vi "load.vi"(8 "error in (no error)":errorcluster, 9 "page":i32, 10 "Path":path, 11 "Image in":refnum<class "Image.lvclass">) -> (0 "error out":errorcluster, 1 "Path out":path, 2 "cancelled?":bool, 3 "Image out":refnum<class "Image.lvclass">)   [LabVIEW 2010, in "Image.lvclass"]
uses:
  Image.lvclass
  storage_mode.ctl
  <vilib>/regexp/Match Regular Expression.xnode
  XMLElement/XMLElement/XMLElement.lvclass
  enumerations/unit.ctl
  ErrorController/ErrorController/class_data.vi
  libraries/TIFFManagement/TIFFManagement.lvlib
  ErrorController/ErrorController/ErrorController.lvclass
panel:
  out "Intensity Graph":u32[][](graph)
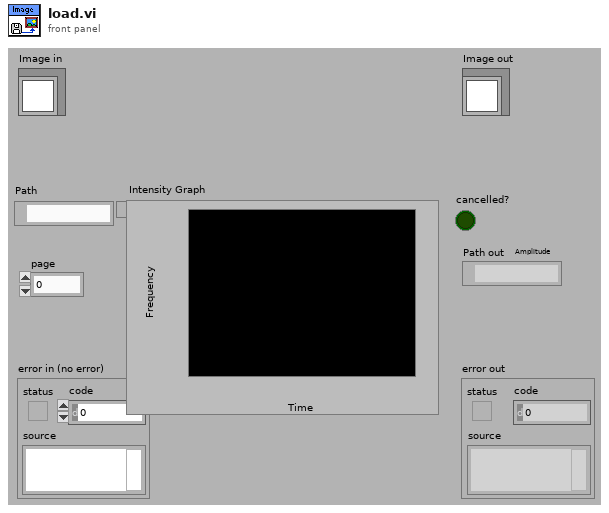
[diagram p1: front panel]
types:
  T1 = typedef "Image.lvclass/storage_mode.ctl" = enum16{"RAM", "disk"}
  T2 = typedef "Image Type" = u32
  T3 = typedef "IMAQ Image.ctl" = refnum<image>
  T4 = typedef "Image.lvclass/unit.ctl" = enum16{"um", "s"}
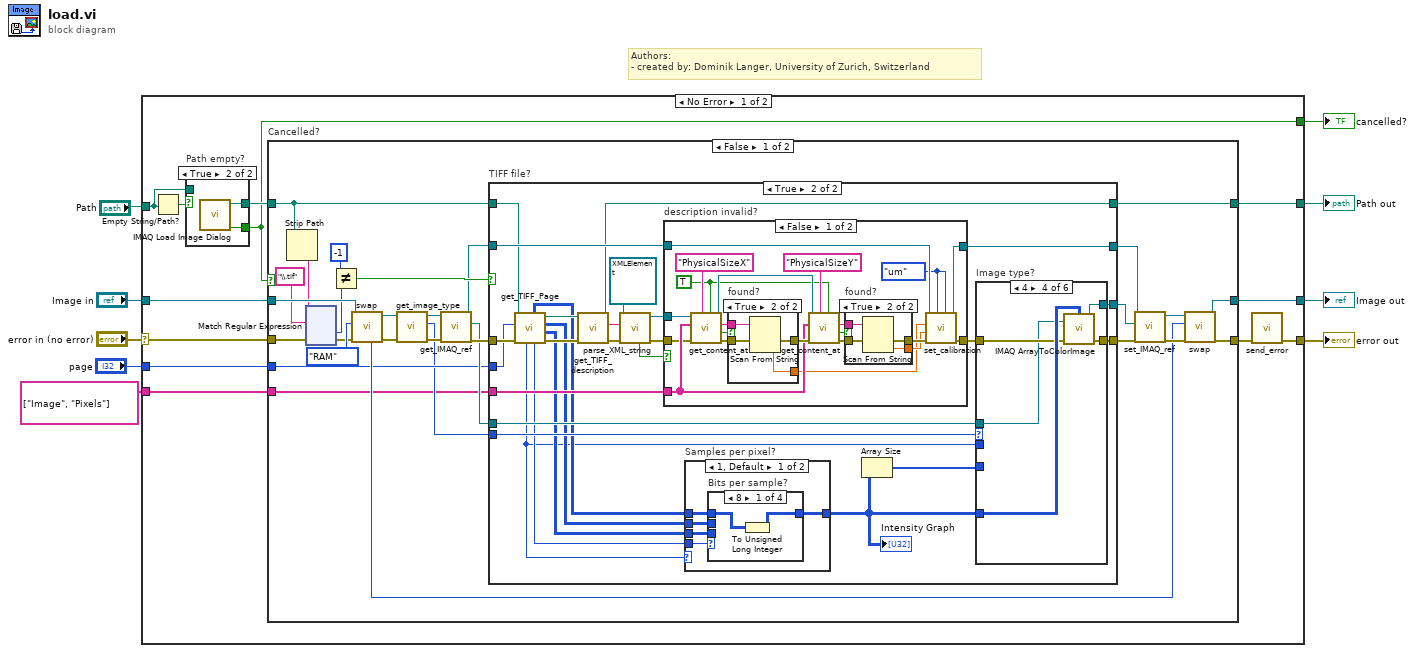
[diagram p0: block diagram]
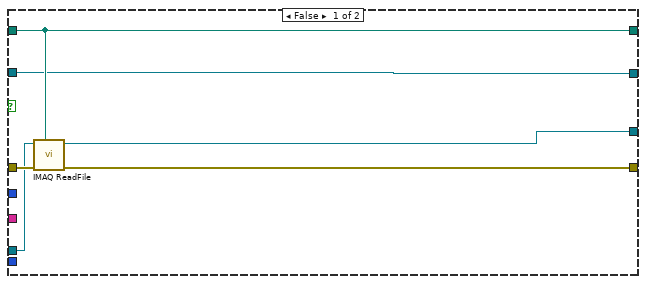
[diagram p2: hidden frame]
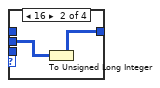
[diagram p3: hidden frame]
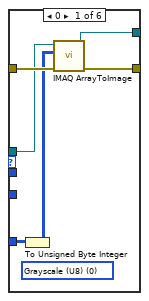
[diagram p10: hidden frame]
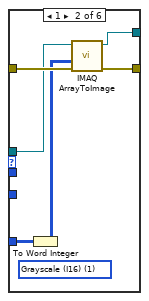
[diagram p11: hidden frame]
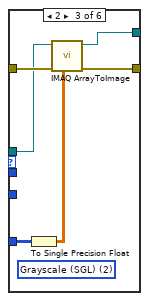
[diagram p12: hidden frame]
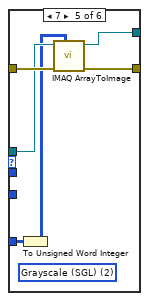
[diagram p13: hidden frame]
diagram:
  # "Authors: \n- created by: Dominik Langer, University of Zurich, Switzerland"
  n1 = case shown="No Error" "error in (no error)" {
    selector: "error in (no error)" -> [w18 w276]
    tunnel: [w11 w276] -> w8
    tunnel: [w20 w275] -> w6
    tunnel: "Image in" -> [w19 w275]
    tunnel: "Path" -> [w17 _]
    tunnel: [w15 _] -> w5
    tunnel: [w14 _] -> w4
    tunnel: "page" -> [w13 _]
    tunnel: string[] ["Image", "Pixels"] ("key chain") -> [w12 _]
    frame No Error {
      n2 = Empty String/Path?(string/path=w17) -> (empty?=w16:bool)
      n3 = case "Path empty?" shown="True" w16 {
        tunnel: [w272 w274] -> w21
        tunnel: w17 -> [w272 _]
        tunnel: [_ w273] -> w15
        frame False {
        }
        frame True {
          n4 = call "IMAQ Load Image Dialog"() -> ("Cancelled?"=w273:bool, "Path"=w274:path)  [unwired: 7 in, 3 out]
        }
      }
      n5 = case "Cancelled?" shown="False" w15 {
        tunnel: w21 -> [w47 _]
        tunnel: [w50 w271] -> w10
        tunnel: [w49 w270] -> w20
        tunnel: w19 -> [w48 w270]
        tunnel: w18 -> [w27 w271]
        tunnel: [w36 _] -> w14
        tunnel: w13 -> [w35 _]
        tunnel: w12 -> [w22 _]
        frame False {
          n6 = Strip Path(path=w47) -> (name=w25:string)  [unwired: 1 out]
          n7 = xnode "Match Regular Expression"("input string"=w25, "regular expression"="\\.tif", "error in"=w27) -> ("offset past match"=w23:i32, "error out"=w26:errorcluster)  [unwired: 3 in, 3 out]
          n8 = Not Equal?(x=-1, y=w23) -> (x != y?=w37:bool)
          n9 = call-dynamic "swap.vi"("error in (no error)"=w26, "storage type target"=storage_mode."RAM", "Image in"=w48) -> ("error out"=w34:errorcluster, "Image out"=w33:refnum<class "Image.lvclass">, "previous storage mode"=w39:T1)  [unwired: 6 out]
          n10 = call-dynamic "get_image_type.vi"("error in (no error)"=w34, "Image.lvclass in"=w33) -> ("error out"=w32:errorcluster, "Image Type"=w30:T2, "Image.lvclass out"=w31:refnum<class "Image.lvclass">)  [unwired: 6 in, 1 out]
          n11 = call-dynamic "get_IMAQ_ref.vi"("error in (no error)"=w32, "Image.lvclass in"=w31) -> ("error out"=w43:errorcluster, "Image"=w42:T3, "Image.lvclass out"=w29:refnum<class "Image.lvclass">)  [unwired: 7 out]
          n12 = case "TIFF file?" shown="True" w37 {
            tunnel: w47 -> [w163 w186]
            tunnel: [w167 w189] -> w45
            tunnel: [w166 w194] -> w44
            tunnel: w43 -> [w165 w187]
            tunnel: w42 -> [w164 w193]
            tunnel: [w163 w182] -> w36
            tunnel: w35 -> [_ w185]
            tunnel: w30 -> [_ w192]
            tunnel: w29 -> [w162 w191]
            tunnel: [w162 w190] -> w28
            tunnel: w22 -> [_ w181]
            frame False {
              n13 = call "IMAQ ReadFile"("File Path"=w163, "error in (no error)"=w165, "Image"=w164) -> ("error out"=w167:errorcluster, "Image Out"=w166:T3)  [unwired: 2 in, 5 out]
            }
            frame True {
              n14 = call "get_TIFF_Page.vi"("error in (no error)"=w187, "page"=w185, "path in"=w186) -> ("error out"=w184:errorcluster, "data 32bit"=w178:u32[][], "data 16bit"=w180:u16[][], "path out"=w183:path, "bits per sample"=w177:u16, "data 8bit"=w179:u8[][], "samples per pixel"=w176:i32)  [unwired: 2 in]
              n15 = call "get_TIFF_description.vi"("error in (no error)"=w184, "path in"=w183) -> ("error out"=w172:errorcluster, "description"=w173:string, "path out"=w182:path)  [unwired: 6 in, 1 out]
              n16 = call "parse_XML_string.vi"("error in (no error)"=w172, "XML string"=w173, "Element in"=refnum<class "XMLElement.lvclass"> refnum ("XMLElement.lvclass")) -> ("error out"=w171:errorcluster, "Element out"=w168:refnum<class "XMLElement.lvclass">, "header empty or invalid XML?"=w169:bool)  [unwired: 6 in]
              n17 = case "description invalid?" shown="False" w169 {
                tunnel: w191 -> [w226 w238]
                tunnel: [w225 w238] -> w190
                tunnel: [w223 w237] -> w188
                tunnel: w171 -> [w207 w237]
                tunnel: w181 -> [w214 _]
                tunnel: w168 -> [w206 _]
                frame False {
                  w211 = TRUE
                  w224 = unit."um" ("x unit")
                  n18 = call "get_content_at.vi"("ignore IDs"=w211, "attribute name"="PhysicalSizeX", "error in (no error)"=w207, "key chain"=w214, "Element in"=w206) -> ("error out"=w221:errorcluster, "found?"=w210:bool, "string"=w219:string, "Element out"=w222:refnum<class "XMLElement.lvclass">)  [unwired: 3 in]
                  n19 = case "found?" shown="True" w210 {
                    tunnel: w221 -> [w232 w236]
                    tunnel: [w232 w235] -> w220
                    tunnel: [_ w234] -> w209
                    tunnel: w219 -> [_ w233]
                    frame False {
                    }
                    frame True {
                      n20 = Scan From String(input string=w233, error in=w236) -> (error out=w235:errorcluster, output 1=w234:dbl)  [unwired: 3 in, 2 out]
                    }
                  }
                  n21 = call "get_content_at.vi"("ignore IDs"=w211, "attribute name"="PhysicalSizeY", "error in (no error)"=w220, "key chain"=w214, "Element in"=w222) -> ("error out"=w218:errorcluster, "found?"=w208:bool, "string"=w216:string)  [unwired: 3 in, 1 out]
                  n22 = case "found?" shown="True" w208 {
                    tunnel: w218 -> [w227 w231]
                    tunnel: [w227 w230] -> w217
                    tunnel: w216 -> [_ w229]
                    tunnel: [_ w228] -> w215
                    frame False {
                    }
                    frame True {
                      n23 = Scan From String(input string=w229, error in=w231) -> (error out=w230:errorcluster, output 1=w228:dbl)  [unwired: 3 in, 2 out]
                    }
                  }
                  n24 = call "set_calibration.vi"("y unit"=w224, "x unit"=w224, "error in (no error)"=w217, "y"=w215, "x"=w209, "Image in"=w226) -> ("error out"=w223:errorcluster, "Image out"=w225:refnum<class "Image.lvclass">)  [unwired: 4 in]
                }
                frame True {
                }
              }
              n25 = case "Samples per pixel?" shown="1, Default" w176 {
                tunnel: w180 -> [w195 _]
                tunnel: w179 -> [w198 _]
                tunnel: w178 -> [w196 w205]
                tunnel: [w197 w205] -> w175
                tunnel: w177 -> [w199 _]
                frame 1, Default {
                  n26 = case "Bits per sample?" shown="8" w199 {
                    tunnel: w198 -> [w201 _ _ _]
                    tunnel: [w200 w203 w204 _] -> w197
                    tunnel: w196 -> [_ _ w204 _]
                    tunnel: w195 -> [_ w202 _ _]
                    frame 8 {
                      n27 = To Unsigned Long Integer(number=w201) -> (unsigned 32bit integer=w200:u32[][])
                    }
                    frame 16 {
                      n28 = To Unsigned Long Integer(number=w202) -> (unsigned 32bit integer=w203:u32[][])
                    }
                    frame 32 {
                    }
                    frame Default {
                    }
                  }
                }
                frame 3 {
                }
              }
              "Intensity Graph" <- w175
              n29 = Array Size(array=w175) -> (size(s)=w174:i32[])
              n30 = case "Image type?" shown="4" w192 {
                tunnel: w188 -> [w243 w250 w255 w260 w267 w268]
                tunnel: [w241 w249 w252 w258 w266 w268] -> w189
                tunnel: w175 -> [w244 w246 w256 w261 w263 _]
                tunnel: [w240 w248 w251 w257 w265 w269] -> w194
                tunnel: w193 -> [w242 w247 w254 w259 w264 w269]
                tunnel: w176 -> [_ _ _ _ _ _]
                tunnel: w174 -> [_ _ _ _ _ _]
                frame 0 {
                  (unwired) T2 0 items=["Grayscale (U8)", "Grayscale (I16)", "Grayscale (SGL)", "Complex (CSG)", "RGB (U32)", "HSL (U32)", "RGB (U64)", "Grayscale (U16)"] ("Image Type")
                  n31 = To Unsigned Byte Integer(number=w244) -> (unsigned 8bit integer=w239:u8[][])
                  n32 = call "IMAQ ArrayToImage"("error in (no error)"=w243, "Image Pixels (U8)"=w239, "Image"=w242) -> ("error out"=w241:errorcluster, "Image Out"=w240:T3)  [unwired: 7 in]
                }
                frame 1 {
                  (unwired) T2 1 items=["Grayscale (U8)", "Grayscale (I16)", "Grayscale (SGL)", "Complex (CSG)", "RGB (U32)", "HSL (U32)", "RGB (U64)", "Grayscale (U16)"] ("Image Type")
                  n33 = To Word Integer(number=w246) -> (16bit integer=w245:i16[][])
                  n34 = call "IMAQ ArrayToImage"("error in (no error)"=w250, "Image Pixels (I16)"=w245, "Image"=w247) -> ("error out"=w249:errorcluster, "Image Out"=w248:T3)  [unwired: 7 in]
                }
                frame 2 {
                  (unwired) T2 2 items=["Grayscale (U8)", "Grayscale (I16)", "Grayscale (SGL)", "Complex (CSG)", "RGB (U32)", "HSL (U32)", "RGB (U64)", "Grayscale (U16)"] ("Image Type")
                  n35 = To Single Precision Float(number=w256) -> (single precision float=w253:sgl[][])
                  n36 = call "IMAQ ArrayToImage"("Image Pixels (Float)"=w253, "error in (no error)"=w255, "Image"=w254) -> ("error out"=w252:errorcluster, "Image Out"=w251:T3)  [unwired: 7 in]
                }
                frame 4 {
                  n37 = call "IMAQ ArrayToColorImage"("Image Pixels (U32)"=w261, "Image"=w259, "error in (no error)"=w260) -> ("Image Out"=w257:T3, "error out"=w258:errorcluster)  [unwired: 2 in]
                }
                frame 7 {
                  (unwired) T2 2 items=["Grayscale (U8)", "Grayscale (I16)", "Grayscale (SGL)", "Complex (CSG)", "RGB (U32)", "HSL (U32)", "RGB (U64)", "Grayscale (U16)"] ("Image Type")
                  n38 = To Unsigned Word Integer(number=w263) -> (unsigned 16bit integer=w262:u16[][])
                  n39 = call "IMAQ ArrayToImage"("Image Pixels (U16)"=w262, "error in (no error)"=w267, "Image"=w264) -> ("error out"=w266:errorcluster, "Image Out"=w265:T3)  [unwired: 7 in]
                }
                frame Default {
                }
              }
            }
          }
          n40 = call-dynamic "set_IMAQ_ref.vi"("error in (no error)"=w45, "Image"=w44, "Image.lvclass in"=w28) -> ("error out"=w40:errorcluster, "Image.lvclass out"=w41:refnum<class "Image.lvclass">)  [unwired: 7 out]
          n41 = call-dynamic "swap.vi"("error in (no error)"=w40, "storage type target"=w39, "Image in"=w41) -> ("error out"=w50:errorcluster, "Image out"=w49:refnum<class "Image.lvclass">)  [unwired: 7 out]
        }
        frame True {
        }
      }
      n42 = call "send_error.vi"("error in (no error)"=w10) -> ("error out"=w11:errorcluster)  [unwired: 10 in]
    }
    frame Error {
    }
  }
  "error out" <- w8
  "Image out" <- w6
  "cancelled?" <- w5
  "Path out" <- w4
